vi "ConfigureTrigger.vi"(8 "error in (no error)":errorcluster, 11 "NIScope in":refnum<class "NIScope.lvclass">) -> (0 "error out":errorcluster, 3 "NIScope out":refnum<class "NIScope.lvclass">)   [LabVIEW 2018, in "ScopePlugins.lvlib" / "NIScope.lvclass"]
uses:
  NIScope.lvclass
  Y:/Projects/PMUCal/Modules/Scope/ScopePlugins/ScopePluginBaseClass/ScopePluginsBase.lvclass
  ScopePluginBaseClass/ScopePluginsBase.lvclass/ScopePluginsBase.ctl
  <instrlib>/niScope/Controls/niScope trigger coupling.ctl
  <instrlib>/niScope/Controls/niScope trigger slope.ctl
  ScopePluginBaseClass/Accessors/Read Trigger.vi
  ScopePluginBaseClass/Accessors/Read Channels.vi
  ScopePluginBaseClass/Accessors/Write Channels.vi
  <vilib>/Utility/error.llb/Error Cluster From Error Code.vi
  <instrlib>/niScope/Configure/Trigger/niScope Configure Trigger Digital.vi
  <instrlib>/niScope/Configure/Trigger/niScope Configure Trigger Window.vi
  <instrlib>/niScope/Configure/Trigger/niScope Configure Trigger Hysteresis.vi
  <instrlib>/niScope/Configure/Trigger/niScope Configure Video Trigger.vi
  <instrlib>/niScope/Configure/Trigger/niScope Configure Trigger Immediate.vi
  <instrlib>/niScope/Configure/Trigger/niScope Configure Trigger Software.vi
  <vilib>/ErrorRing/Error Ring.xnode
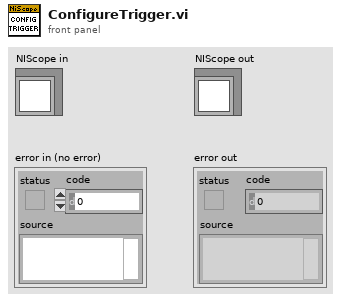
[diagram p1: front panel]
types:
  T1 = typedef "ScopePlugins.lvlib/Channels.ctl" = cluster{"Count":i32, "ChannelArray":T2[]}
  T2 = typedef "ScopePlugins.lvlib/Channel.ctl" = cluster{"Enabled":bool, "Name":string, "InputImpedance":dbl, "InputFreqMax":dbl, "ProbeAttn":dbl, "Coupling":enum16{"AC", "DC", "GND"}, "Offset":dbl, "Range":dbl, "Handle":string, "Connected":bool}
  T3 = typedef "ScopePlugins.lvlib/Trigger.ctl" = cluster{"Coupling":enum16{"AC", "DC", "LF Reject", "HF Reject", "Noise Reject"}, "Holdoff":dbl, "Level":dbl, "Slope":enum16{"Negative", "Positive"}, "Source":string, "Type":enum16{"Edge", "Width", "Runt", "Glitch", "TV", "Immediate", "AC Line"}}
  T4 = enum16{"AC", "DC", "LF Reject", "HF Reject", "Noise Reject"}
  T5 = enum16{"Edge", "Width", "Runt", "Glitch", "TV", "Immediate", "AC Line"}
  T6 = typedef "niScope trigger coupling.ctl" = u16
  T7 = typedef "niScope trigger slope.ctl" = i32
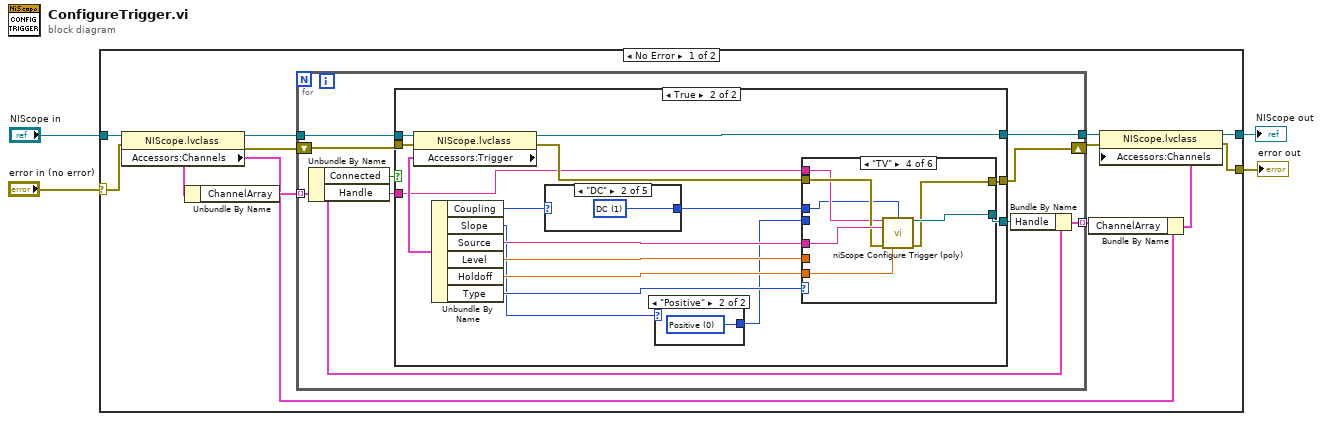
[diagram p0: block diagram]
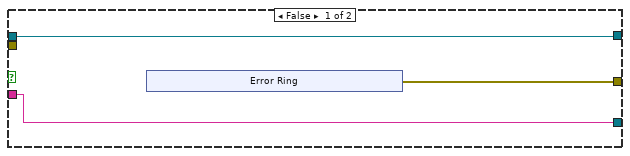
[diagram p2: hidden frame]
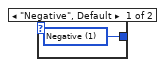
[diagram p3: hidden frame]
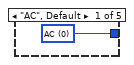
[diagram p4: hidden frame]
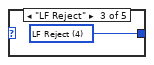
[diagram p5: hidden frame]
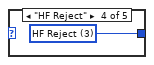
[diagram p6: hidden frame]
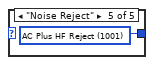
[diagram p7: hidden frame]
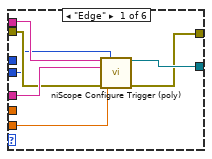
[diagram p8: hidden frame]
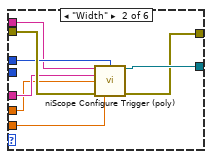
[diagram p9: hidden frame]
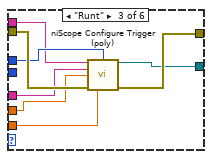
[diagram p10: hidden frame]
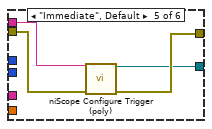
[diagram p11: hidden frame]
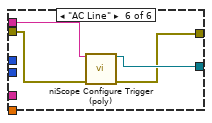
[diagram p12: hidden frame]
diagram:
  n1 = case shown="No Error" "error in (no error)" {
    selector: "error in (no error)" -> [w15 w95]
    tunnel: "NIScope in" -> [w16 w96]
    tunnel: [w10 w96] -> w2
    tunnel: [w8 w95] -> w1
    frame No Error {
      n2 = property class="NIScope.lvclass"(reference=w16, error in=w15) -> (reference out=w12:refnum<class "NIScope.lvclass">, error out=w11:errorcluster, "Accessors:Channels"=w7:T1)
      n3 = Unbundle By Name(w7) -> ("ChannelArray"=w13:T2[])
      n4 = for {
        tunnel: [w25] -> w14
        tunnel: w13 -> [w20] mode=indexing
        tunnel: w12 -> [w24]
        shift-right: [w21] -> w9
        shift-left: w11 -> [w23]
        tunnel: [w19] -> w6 mode=indexing
        n5 = Unbundle By Name(w20) -> ("Connected"=w17:bool, "Handle"=w22:string)
        n6 = case shown="True" w17 {
          tunnel: w24 -> [w28 w49]
          tunnel: [w28 w44] -> w25
          tunnel: [w27 w43] -> w21
          tunnel: w23 -> [_ w39]
          tunnel: w22 -> [w26 w38]
          tunnel: [w26 w37] -> w18
          frame False {
            n7 = xnode "Error Ring"() -> ("error out"=w27:errorcluster)
          }
          frame True {
            n8 = property class="NIScope.lvclass"(reference=w49, error in=w39) -> (reference out=w44:refnum<class "NIScope.lvclass">, error out=w45:errorcluster, "Accessors:Trigger"=w40:T3)
            n9 = Unbundle By Name(w40) -> ("Coupling"=w42:T4, "Slope"=w35:enum16{"Negative", "Positive"}, "Source"=w36:string, "Level"=w47:dbl, "Holdoff"=w46:dbl, "Type"=w48:T5)
            n10 = case shown="\"DC\"" w42 {
              tunnel: [w52 w53 w54 w55 w56] -> w41
              frame "AC", Default {
                w52 = T6 0 items=["AC"=0, "DC"=1, "HF Reject"=3, "LF Reject"=4, "AC Plus HF Reject"=1001] ("trigger coupling")
              }
              frame "DC" {
                w53 = T6 1 items=["AC"=0, "DC"=1, "HF Reject"=3, "LF Reject"=4, "AC Plus HF Reject"=1001] ("trigger coupling")
              }
              frame "LF Reject" {
                w54 = T6 4 items=["AC"=0, "DC"=1, "HF Reject"=3, "LF Reject"=4, "AC Plus HF Reject"=1001] ("trigger coupling")
              }
              frame "HF Reject" {
                w55 = T6 3 items=["AC"=0, "DC"=1, "HF Reject"=3, "LF Reject"=4, "AC Plus HF Reject"=1001] ("trigger coupling")
              }
              frame "Noise Reject" {
                w56 = T6 1001 items=["AC"=0, "DC"=1, "HF Reject"=3, "LF Reject"=4, "AC Plus HF Reject"=1001] ("trigger coupling")
              }
            }
            n11 = case shown="\"Positive\"" w35 {
              tunnel: [w50 w51] -> w34
              frame "Negative", Default {
                w50 = T7 1 items=["Positive", "Negative"] ("trigger slope")
              }
              frame "Positive" {
                w51 = T7 0 items=["Positive", "Negative"] ("trigger slope")
              }
            }
            n12 = case shown="\"TV\"" w48 {
              tunnel: w36 -> [w63 w68 w76 w85 _ _]
              tunnel: w47 -> [_ w64 w72 _ _ _]
              tunnel: w46 -> [w62 w67 w74 w84 _ _]
              tunnel: [w61 w71 w77 w86 w88 w92] -> w37
              tunnel: w45 -> [w60 w70 w79 w83 w90 w94]
              tunnel: [w59 w69 w78 w82 w89 w91] -> w43
              tunnel: w41 -> [_ w66 w75 w80 _ _]
              tunnel: w38 -> [w58 w65 w73 w81 w87 w93]
              tunnel: w34 -> [w57 _ _ _ _ _]
              frame "Edge" {
                n13 = call-poly <instrlib>:"niScope Configure Trigger (poly).vi"("instrument handle"=w58, "trigger slope"=w57, "trigger source"=w63, "error in"=w60, "trigger holdoff"=w62) -> ("instrument handle out"=w61:refnum<k15>, "error out"=w59:errorcluster)  [unwired: 9 in]
              }
              frame "Width" {
                n14 = call-poly <instrlib>:"niScope Configure Trigger (poly).vi"("instrument handle"=w65, "trigger coupling"=w66, "trigger source"=w68, "low level"=w64, "error in"=w70, "trigger holdoff"=w67) -> ("instrument handle out"=w71:refnum<k15>, "error out"=w69:errorcluster)  [unwired: 8 in]
              }
              frame "Runt" {
                n15 = call-poly <instrlib>:"niScope Configure Trigger (poly).vi"("instrument handle"=w73, "trigger coupling"=w75, "trigger source"=w76, "trigger level"=w72, "error in"=w79, "trigger holdoff"=w74) -> ("instrument handle out"=w77:refnum<k15>, "error out"=w78:errorcluster)  [unwired: 8 in]
              }
              frame "TV" {
                n16 = call-poly <instrlib>:"niScope Configure Trigger (poly).vi"("instrument handle"=w81, "trigger coupling"=w80, "trigger source"=w85, "error in"=w83, "trigger holdoff"=w84) -> ("instrument handle out"=w86:refnum<k15>, "error out"=w82:errorcluster)  [unwired: 9 in]
              }
              frame "Immediate", Default {
                n17 = call-poly <instrlib>:"niScope Configure Trigger (poly).vi"("instrument handle"=w87, "error in"=w90) -> ("instrument handle out"=w88:refnum<k15>, "error out"=w89:errorcluster)  [unwired: 12 in]
              }
              frame "AC Line" {
                n18 = call-poly <instrlib>:"niScope Configure Trigger (poly).vi"("instrument handle"=w93, "error in"=w94) -> ("instrument handle out"=w92:refnum<k15>, "error out"=w91:errorcluster)  [unwired: 12 in]
              }
            }
          }
        }
        n19 = Bundle By Name(cluster=w20, "Handle"=w18) -> (w19:T2)
      }
      n20 = Bundle By Name(cluster=w7, "ChannelArray"=w6) -> (w5:T1)
      n21 = property class="NIScope.lvclass"(reference=w14, error in=w9, "Accessors:Channels"=w5) -> (reference out=w10:refnum<class "NIScope.lvclass">, error out=w8:errorcluster)
    }
    frame Error {
    }
  }
  "error out" <- w1
  "NIScope out" <- w2
